vi "Close.vi"(8 "error in (no error)":errorcluster, 11 "Modbus master in":refnum<class "Modbus Master.lvclass">) -> (0 "error out":errorcluster)   [LabVIEW 2015, in "Modbus Master.lvclass"]
doc: "Closes and destroys a Modbus master instance."
uses:
  <vilib>/Modbus/master/Modbus Master.lvclass
  <vilib>/Modbus/master/Modbus Master.lvclass/Modbus Master.ctl
  <vilib>/Modbus/subvis/Protocol/Interfaces/Network Master/Network Master.lvclass
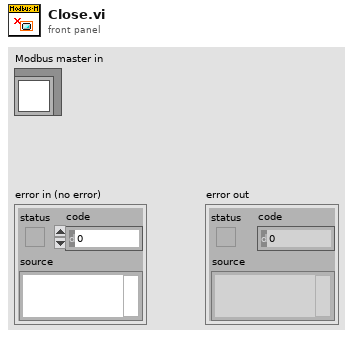
[diagram p1: front panel]
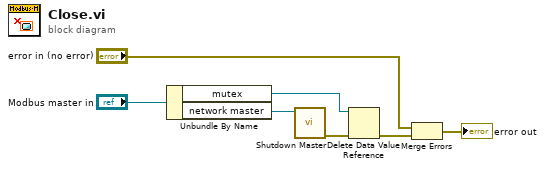
[diagram p0: block diagram]
diagram:
  n1 = Unbundle By Name("Modbus master in") -> ("mutex"=w5:refnum<data-value>, "network master"=w6:refnum<class "Network Master.lvclass">)
  n2 = call-dynamic "Shutdown Master.vi"("network master in"=w6) -> ("error out"=w4:errorcluster)  [unwired: 9 in, 1 out]
  n3 = Delete Data Value Reference(data value reference=w5, error in=w4) -> (error out=w3:errorcluster)  [unwired: 1 out]
  n4 = Merge Errors("error in (no error)", w3) -> (→"error out":errorcluster)
